vi "Load Single Texture From ANI.vi"(8 "error in (no error)":errorcluster, 10 "Index":i32, 11 "Star ANI File":path) -> (0 "error out":errorcluster, 2 "Hotspot":T1, 3 "Name In Cache":string)   [LabVIEW 2021, in "Star.lvclass"]
uses:
  Star/Star.lvclass
  Star/Star.lvclass/Star.ctl
  <userlib>/_OpenG.lib/string/string.llb/openg_string.lvlib
  LabSDL2/Source/Libraries/SDL2 Utility/Point (I32).ctl
  LabSDL2/Source/Libraries/SDL2 Utility/SDL2 Utility.lvlib
  Resource Manager/Resource Manager.lvclass
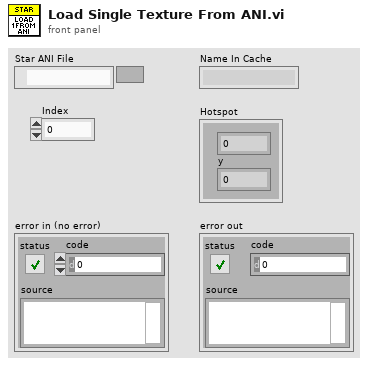
[diagram p1: front panel]
types:
  T1 = typedef "SDL2 Utility.lvlib/Point (I32).ctl" = cluster{"x":i32, "y":i32}
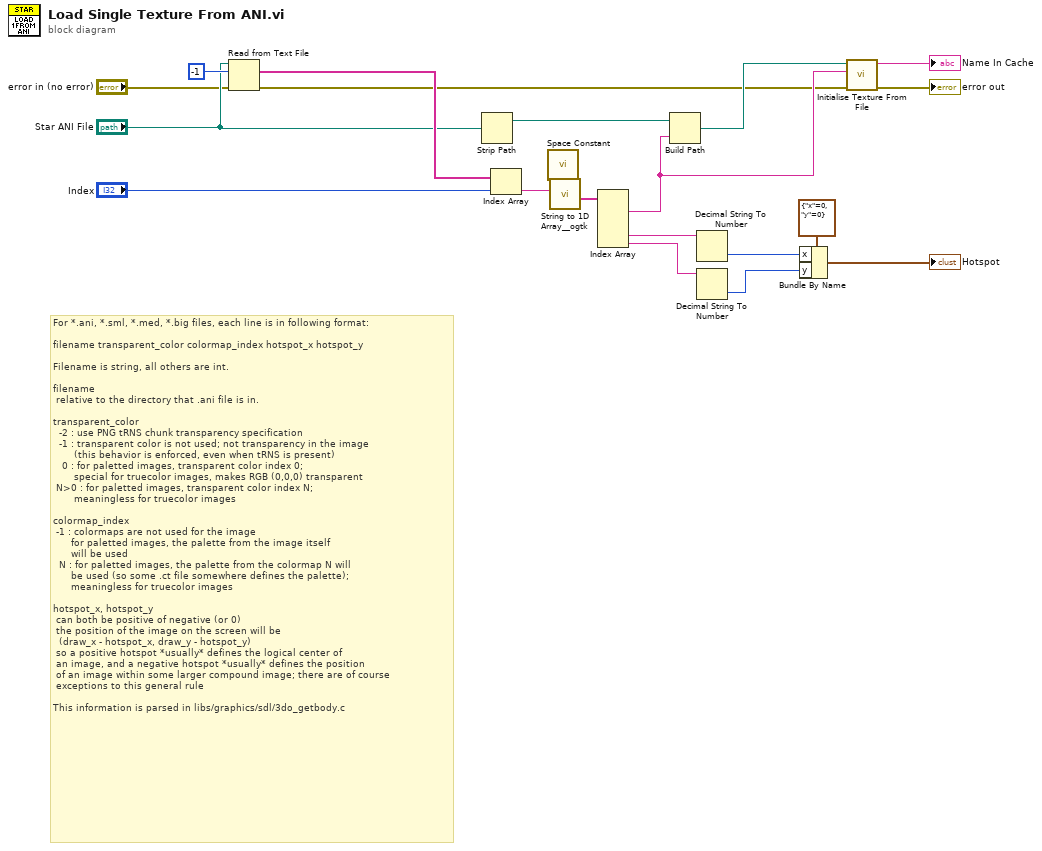
[diagram p0: block diagram]
diagram:
  # "For *.ani, *.sml, *.med, *.big files, each line is in following format:\n\nfilename transparent_color colormap_index hotspot_x hotspot_y\n\nFilename is string, all others are int.\n\nfilename\n\trelative to the directory that .ani file is in.\n\ntransparent_color\n\t -2 : use PNG tRNS chunk transparency specification\n\t -1 : transparent color is not used; not transparency in the image\n\t      (this behavior is enforced, even when tRNS is present)\n\t  0 : for paletted images, transparent color index 0;\n\t      special for truecolor images, makes RGB (0,0,0) transparent\n\tN>0 : for paletted images, transparent color index N;\n\t      meaningless for truecolor images\n\ncolormap_index\n\t-1 : colormaps are not used for the image\n\t     for paletted images, the palette from the image itself\n\t     will be used\n\t N : for paletted images, the palette from the colormap N will\n\t     be used (so some .ct file somewhere defines the palette);\n\t     meaningless for truecolor images\n\nhotspot_x, hotspot_y\n\tcan both be positive of negative (or 0)\n\tthe position of the image on the screen will be\n\t\t(draw_x - hotspot_x, draw_y - hotspot_y)\n\tso a positive hotspot *usually* defines the logical center of\n\tan image, and a negative hotspot *usually* defines the position\n\tof an image within some larger compound image; there are of course\n\texceptions to this general rule\n\nThis information is parsed in libs/graphics/sdl/3do_getbody.c"
  n1 = Read from Text File(file (use dialog)="Star ANI File", count=-1, error in="error in (no error)") -> (text=w19:string[], error out=w2:errorcluster)  [unwired: 1 in, 2 out]
  n2 = Strip Path(path="Star ANI File") -> (stripped path=w7:path)  [unwired: 1 out]
  n3 = Index Array(array=w19, index="Index") -> (element=w20:string)
  n4 = call <vilib>:"Space Constant.vi"() -> ("String"=w12:string)
  n5 = call <userlib>:"String to 1D Array__ogtk.vi"("delimiter (Tab)"=w12, "string"=w20) -> ("Array of Strings"=w13:string[])  [unwired: 9 in]
  n6 = Index Array(array=w13) -> (element #1=w5:string, element #4=w14:string, element #5=w15:string)  [unwired: 5 in, 2 out]
  n7 = Build Path(base path=w7, name or relative path=w5) -> (appended path=w6:path)
  n8 = Decimal String To Number(string=w14) -> (number=w10:i32)  [unwired: 2 in, 1 out]
  n9 = Decimal String To Number(string=w15) -> (number=w9:i32)  [unwired: 2 in, 1 out]
  n10 = Bundle By Name(cluster=T1 {"x"=0, "y"=0} ("Point"), "x"=w10, "y"=w9) -> (→"Hotspot":T1)
  n11 = call "Initialise Texture From File.vi"("error in (no error)"=w2, "Name"=w5, "File"=w6) -> ("error out"=→"error out":errorcluster, "Name In Cache"=→"Name In Cache":string)  [unwired: 7 in]
